vi "ziConnectDevice.vi"(7 "Device Interface Params (\"\")":string, 8 "Error In":errorcluster, 9 "Device Interface":string, 10 "Device Serial":string, 11 "Handle In":T1 {"Handle" format="0x%08x"; "Conn" format="0x%08x"}) -> (0 "Error Out":errorcluster, 3 "Handle Out":T1 {"Handle" format="0x%08x"; "Conn" format="0x%08x"})   [LabVIEW 2009, in "Zurich Instruments LabOne.lvlib"]
uses:
  <instrlib>/Zurich Instruments LabOne/Zurich Instruments LabOne.lvlib
  <instrlib>/Zurich Instruments LabOne/Public/ziTypeHandle.ctl
  <instrlib>/Zurich Instruments LabOne/Private/ziLV64.dll
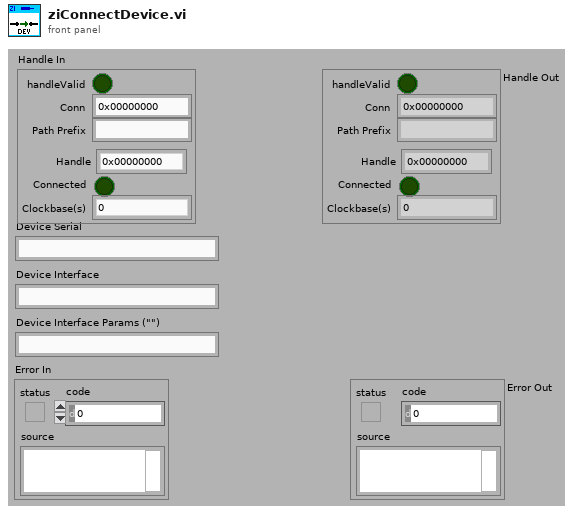
[diagram p1: front panel]
types:
  T1 = typedef "Zurich Instruments LabOne.lvlib/ziTypeHandle.ctl" = cluster{"handleValid":bool, "Conn":u64, "Path Prefix":string, "Handle":u64, "Connected":bool, "Clockbase(s)":dbl}
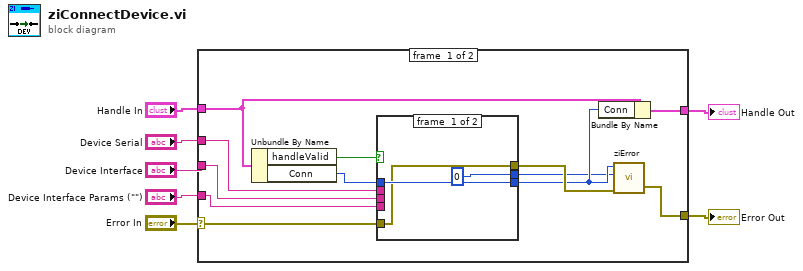
[diagram p0: block diagram]
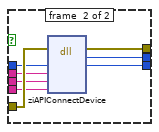
[diagram p2: hidden frame]
diagram:
  n1 = case shown="No Error" "Error In" {
    selector: "Error In" -> [w13 w32]
    tunnel: "Device Interface" -> [w18 _]
    tunnel: [w17 w32] -> w7
    tunnel: [w14 w31] -> w6
    tunnel: "Handle In" -> [w10 w31]
    tunnel: "Device Serial" -> [w12 _]
    tunnel: "Device Interface Params (\"\")" -> [w11 _]
    frame #0 {
      n2 = Unbundle By Name(w10) -> ("handleValid"=w15:bool, "Conn"=w19:u64)
      n3 = case shown="True" w15 {
        tunnel: w13 -> [w21 w30]
        tunnel: w19 -> [w22 w29]
        tunnel: w12 -> [_ w28]
        tunnel: w18 -> [_ w23]
        tunnel: [w21 w27] -> w16
        tunnel: [u32 0 ("return type") w26] -> w8
        tunnel: [w22 w25] -> w9
        tunnel: w11 -> [_ w24]
        frame #0 {
        }
        frame #1 {
          n4 = dll-call lib="C:/Program Files/National Instruments/LabVIEW 2009/instr.lib/Zurich Instruments LabOne/Private/ziLV*.*" fn="ziAPIConnectDevice"(error in=w30, "Conn"=w29, "deviceSerial"=w28, "deviceInterface"=w23, "interfaceParams"=w24) -> (error out=w27:errorcluster, "return type"=w26:u32, "Conn"=w25:u64)  [unwired: 5 in, 1 out]
        }
      }
      n5 = Bundle By Name(cluster=w10, "Conn"=w9) -> (w14:T1)
      n6 = call <instrlib>:"ziError.vi"("Conn"=w9, "ziErrorCode"=w8, "Error In"=w16) -> ("Error Out"=w17:errorcluster)  [unwired: 2 in, 1 out]
    }
    frame #1 {
    }
  }
  "Error Out" <- w7
  "Handle Out" <- w6
